vi "Initialize Interface Global.vi"(8 "error in (no error)":errorcluster, 11 "Interface Parameters":T1) -> (0 "error out":errorcluster)   [LabVIEW 2019, in "FootScan Engine.lvlib"]
uses:
  FootScan Engine.lvlib
  Interface Parameters.ctl
  <userlib>/JUL/Event Message Module/Event Message Library/Event Message.lvlib
panel:
  # "Input"
  # "Output"
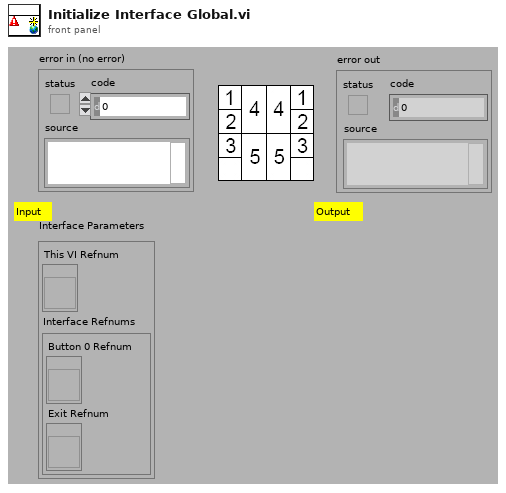
[diagram p1: front panel]
types:
  T1 = typedef "FootScan Engine.lvlib/Interface Parameters.ctl" = cluster{"This VI Refnum":refnum<vi>, "Interface Refnums":cluster{"Button 0 Refnum":refnum<vi>, "Exit Refnum":refnum<vi>}}
  T2 = cluster{"Button 0 Refnum":refnum<vi>, "Exit Refnum":refnum<vi>}
  T3 = typedef "Event Message.lvlib/Event.ctl" = refnum<user-event>
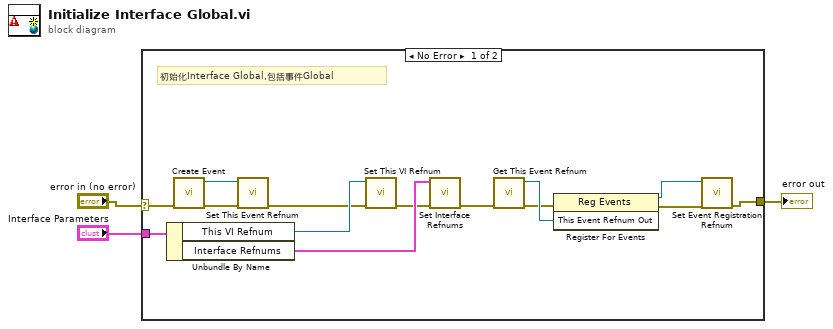
[diagram p0: block diagram]
diagram:
  n1 = case shown="No Error" "error in (no error)" {
    selector: "error in (no error)" -> [w16 w18]
    tunnel: [w10 w18] -> w2
    tunnel: "Interface Parameters" -> [w8 _]
    frame No Error {
      # "初始化Interface Global,包括事件Global"
      n2 = Unbundle By Name(w8) -> ("This VI Refnum"=w6:refnum<vi>, "Interface Refnums"=w7:T2)
      n3 = call <userlib>:"Create Event.vi"("error in (no error)"=w16) -> ("error out"=w15:errorcluster, "Event Out"=w17:T3)  [unwired: 9 in]
      n4 = call "Set This Event Refnum.vi"("error in (no error)"=w15, "This Event Refnum In"=w17) -> ("error out"=w5:errorcluster)  [unwired: 9 in]
      n5 = call "Set This VI Refnum.vi"("error in (no error)"=w5, "This VI Refnum In"=w6) -> ("error out"=w4:errorcluster)  [unwired: 9 in]
      n6 = call "Set Interface Refnums.vi"("error in (no error)"=w4, "Button 0 Refnum"=w7) -> ("error out"=w9:errorcluster)  [unwired: 9 in]
      n7 = call "Get This Event Refnum.vi"("error in (no error)"=w9) -> ("error out"=w13:errorcluster, "This Event Refnum Out"=w14:T3)  [unwired: 9 in]
      n8 = register-events(error in=w13, w14) -> (reference out=w11:refnum<event-registration>, error out=w12:errorcluster)  [unwired: 1 in]
      n9 = call "Set Event Registration Refnum.vi"("error in (no error)"=w12, "Event Registration Refnum in"=w11) -> ("error out"=w10:errorcluster)  [unwired: 9 in]
    }
    frame Error {
    }
  }
  "error out" <- w2
